vi "Gauss fit (SubVI).vi"(6 "parameter bounds":T1={"amp min"=15.0, "amp max"=70000.0, "center min"=5.0, "center max"=83.0, "deviation min"=0.0, "deviation max"=40.0, "offset min"=-100.0, "offset max"=1500.0}, 9 "Array":dbl[](array[numeric])=[97.33333333333333, 95.16666666666667, 93.66666666666667, 91.16666666666667, 96.83333333333333, 97.5, 96.66666666666667, 90.83333333333333, 89.33333333333333, 89.16666666666667, 100.66666666666667, 92.33333333333333, 96.33333333333333, 92.66666666666667, 89.66666666666667, 91.16666666666667, 89.5, 88.16666666666667, 94.66666666666667, 97.66666666666667, 97.83333333333333, 94.16666666666667, 91.83333333333333, 92.66666666666667, 93.83333333333333, 88.83333333333333, 93.16666666666667, 94.0, 94.5, 90.16666666666667, 91.66666666666667, 96.16666666666667, 89.5, 89.66666666666667, 91.83333333333333, 90.33333333333333, 92.66666666666667, 95.33333333333333, 94.83333333333333, 93.0, 94.0, 92.16666666666667, 95.5, 93.16666666666667, 91.83333333333333, 94.83333333333333, 88.83333333333333, 91.5, 96.83333333333333, 93.5, 97.83333333333333, 89.66666666666667, 93.16666666666667, 93.0, 95.33333333333333, 94.5, 90.5, 91.33333333333333, 93.33333333333333, 93.16666666666667, 93.0, 93.16666666666667, 93.33333333333333, 87.33333333333333, 98.0, 92.66666666666667, 95.16666666666667, 96.33333333333333, 87.33333333333333, 96.0, 91.16666666666667, 92.0, 90.5, 88.0, 97.66666666666667, 95.5, 92.33333333333333, 94.33333333333333, 84.5, 90.16666666666667, 91.5, 98.83333333333333, 95.83333333333333, 89.66666666666667, 94.83333333333333, 98.0, 90.0, 104.16666666666667], 10 "initial standard deviation":dbl=4.0, 11 "offset":dbl=100.0) -> (0 "results (a,c,s,r)":dbl[](array[numeric]), 1 "Best Gaussian Fit":dbl[](array[numeric])=[93.13127182309418, 93.13127182309418, 93.13127182309418, 93.13127182309418, 93.13127182309418, 93.13127182309418, 93.13127182309418, 93.13127182309418, 93.13127182309418, 93.13127182309418, 93.13127182309418, 93.13127182309418, 93.13127182309418, 93.13127182309418, 93.13127182309418, 93.13127182309418, 93.13127182309418, 93.13127182309418, 93.13127182309418, 93.13127182309418, 93.13127182309418, 93.13127182309418, 93.13127182309418, 93.13127182309418, 93.13127182309418, 93.13127182309418, 93.13127182309418, 93.13127182309418, 93.13127182309418, 93.13127182309418, 93.13127182309418, 93.13127182309418, 93.13127182309418, 93.13127182309418, 93.13127182309418, 93.13127182309418, 93.13127182309418, 93.13127182309418, 93.13127182309418, 93.13127182309418, 93.13127182309418, 93.13127182309418, 93.13127182309418, 93.13127182309418, 93.13127182309418, 93.13127182309418, 93.13127182309418, 93.13127182309418, 93.13127182309418, 93.13127182309418, 93.13127182309418, 93.13127182309418, 93.13127182309418, 93.13127182309418, 93.13127182309418, 93.13127182309418, 93.13127182309418, 93.13127182309418, 93.13127182309418, 93.13127182309418, 93.13127182309418, 93.13127182309418, 93.13127182309418, 93.13127182309418, 93.13127182309418, 93.13127182309418, 93.13127182309418, 93.13127182309418, 93.13127182309418, 93.13127182309418, 93.13127182309418, 93.13127182309418, 93.13127182309418, 93.13127182309418, 93.13127182309418, 93.13127182309418, 93.13127182309418, 93.13127182309418, 93.13127182309418, 93.13127182309418, 93.13127182309418, 93.13127182309418, 93.13127182309418, 93.13127182309418, 93.13127182309418, 93.13127182309418, 93.13127182309418, 93.13127182309418], 2 "amplitude":dbl=15.0, 3 "center":dbl=74.5883330768061, 4 "standard deviation":dbl, 5 "residue":dbl=10.6253279288955)   [LabVIEW 2018]
uses:
  <vilib>/Analysis/NI_AALPro.lvlib
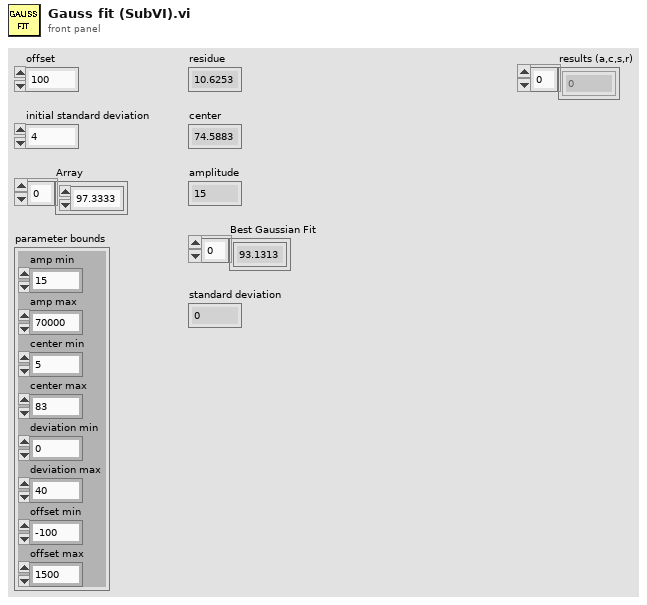
[diagram p1: front panel]
types:
  T1 = cluster{"amp min":dbl, "amp max":dbl, "center min":dbl, "center max":dbl, "deviation min":dbl, "deviation max":dbl, "offset min":dbl, "offset max":dbl}
  T2 = cluster{"initial amplitude":dbl, "initial center":dbl, "initial standard deviation":dbl, "offset":dbl}
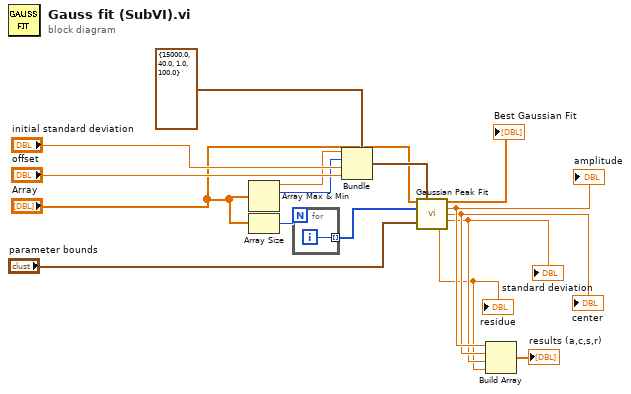
[diagram p0: block diagram]
diagram:
  n1 = Array Max & Min(array="Array") -> (max value=w11:dbl, max index (indices)=w12:i32)  [unwired: 2 out]
  n2 = Array Size(array="Array") -> (size(s)=w15:i32)
  n3 = for {
    N: w15 -> [_]
    tunnel: [w17] -> w8 mode=indexing
    i -> [w17]
  }
  n4 = Bundle(cluster=T2 {"initial amplitude"=15000.0, "initial center"=40.0, "initial standard deviation"=1.0, "offset"=100.0} ("initial guess"), "initial amplitude"=w11, "initial center"=w12, "initial standard deviation"="initial standard deviation", "offset"="offset") -> (w10:T2)
  n5 = call <vilib>:"Gaussian Peak Fit.vi"("Y"="Array", "initial guess"=w10, "X"=w8, "parameter bounds"="parameter bounds") -> ("Best Gaussian Fit"=→"Best Gaussian Fit":dbl[], "amplitude"=w5:dbl, "center"=w4:dbl, "standard deviation"=w3:dbl, "residue"=w2:dbl)  [unwired: 5 in, 2 out]
  "residue" <- w2
  "center" <- w4
  "amplitude" <- w5
  "standard deviation" <- w3
  n6 = Build Array(w5, w4, w3, w2) -> (→"results (a,c,s,r)":dbl[])
